vi "DrawList.vi"(8 "error in (no error)":errorcluster, 9 "Position":T1, 11 "Highscore in":refnum<class "HighscoreDialog.lvclass">) -> (0 "error out":errorcluster, 3 "Highscore out":refnum<class "HighscoreDialog.lvclass">)   [LabVIEW 2019, in "RT_Game.lvlib" / "HighscoreDialog.lvclass"]
uses:
  HighscoreDialog.lvclass
  Engine/Coordinate.ctl
  HighscoreDialog.lvclass/HighscoreDialog.ctl
  Engine/Engine.lvclass
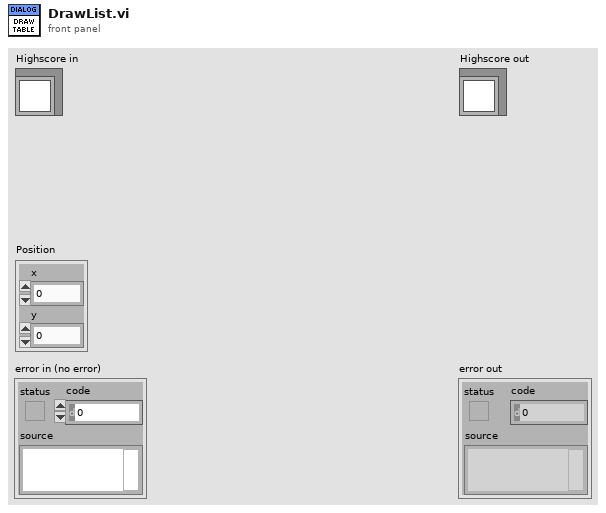
[diagram p1: front panel]
types:
  T1 = typedef "RT_Game.lvlib/Engine.lvclass/Coordinate.ctl" = cluster{"x":dbl, "y":dbl}
  T2 = typedef "RT_Game.lvlib/Highscore.lvclass/HighscoreEntry.ctl" = cluster{"Name":string, "Score":dbl}
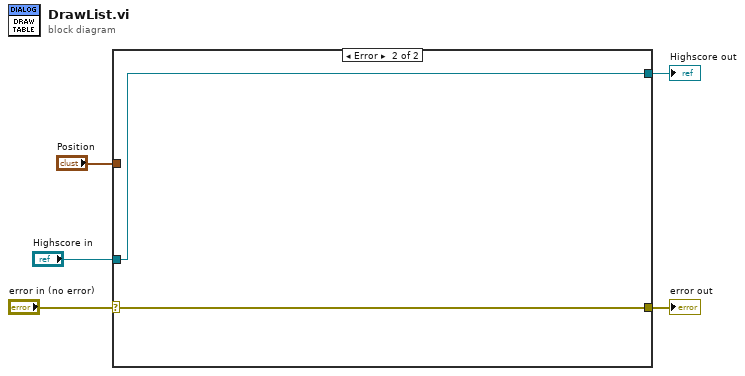
[diagram p0: block diagram]
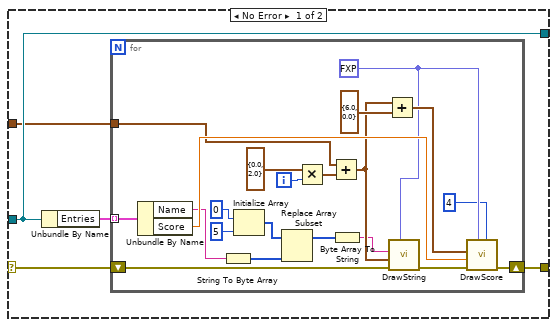
[diagram p2: hidden frame]
diagram:
  n1 = case shown="Error" "error in (no error)" {
    selector: "error in (no error)" -> [w10 w33]
    tunnel: [w9 w33] -> w4
    tunnel: [w8 w32] -> w2
    tunnel: "Highscore in" -> [w8 w32]
    tunnel: "Position" -> [w6 _]
    frame No Error {
      n2 = Unbundle By Name(w8) -> ("Entries"=w7:T2[])
      n3 = for {
        shift-right: [w29] -> w9
        shift-left: w10 -> [w31]
        tunnel: w7 -> [w28] mode=indexing
        tunnel: w6 -> [w26]
        i -> [w18]
        w20 = fxp<+,3,3> 7.0 ("Color (7=white)")
        n4 = Unbundle By Name(w28) -> ("Name"=w14:string, "Score"=w27:dbl)
        n5 = String To Byte Array(string=w14) -> (unsigned byte array=w13:u8[])
        n6 = Initialize Array(u8 0 ("element"), 5 ("dimension size")) -> (w15:u8[])
        n7 = Replace Array Subset(array=w15, new element=w13) -> (w12:u8[])  [unwired: 1 in]
        n8 = Multiply(x=T1 {"x"=0.0, "y"=2.0}, y=w18) -> (x*y=w21:T1)
        n9 = Add(x=w26, y=w21) -> (x+y=w23:T1)
        n10 = Byte Array To String(unsigned byte array=w12) -> (string=w11:string)
        n11 = Add(x=w23, y=T1 {"x"=6.0, "y"=0.0}) -> (x+y=w24:T1)
        n12 = call "DrawString.vi"("Color (7=white)"=w20, "error in (no error)"=w31, "Coordinate"=w23, "String"=w11) -> ("error out"=w30:errorcluster)  [unwired: 7 in]
        n13 = call "DrawScore.vi"("Digits"=4, "Color"=w20, "error in (no error)"=w30, "score"=w27, "position"=w24) -> ("error out"=w29:errorcluster)  [unwired: 6 in]
      }
    }
    frame Error {
    }
  }
  "error out" <- w4
  "Highscore out" <- w2
